vi "Access Privilege_UpdateLoginFile.vi"(8 "error in":errorcluster, 9 "Password":string, 10 "UserID":string, 11 "Cluster_In":T1) -> (0 "error out":errorcluster, 3 "Cluster_In 2":T1)   [LabVIEW 2023, in "GUI.lvlib"]
uses:
  GUI.lvlib
  Typedefs/Access Privilege_Account ManagerAppCluster.ctl
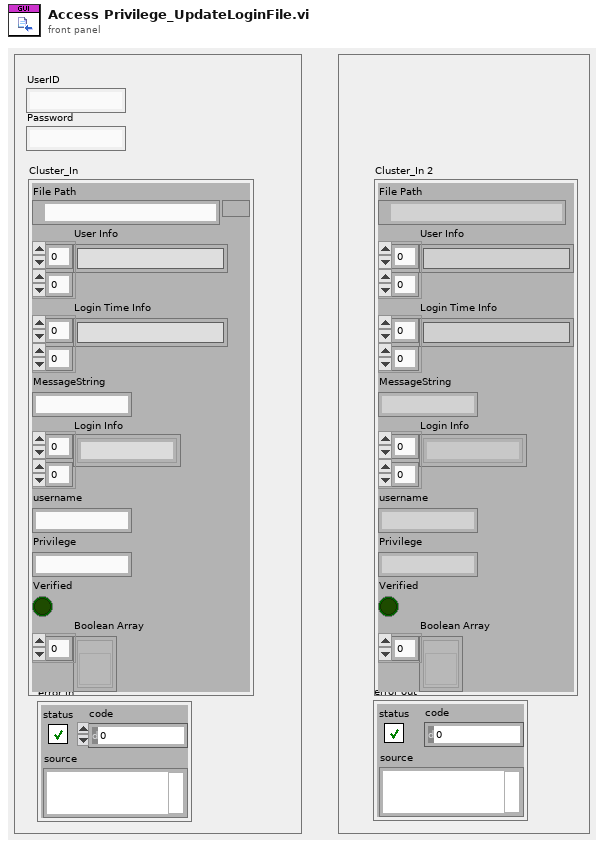
[diagram p1: front panel]
types:
  T1 = typedef "GUI.lvlib/Access Privilege_Account ManagerAppCluster.ctl" = cluster{"File Path":path, "User Info":string[][], "Login Time Info":string[][], "MessageString":string, "Login Info":string[][], "username":string, "Privilege":string, "Verified":bool, "Boolean Array":refnum<vi>[]}
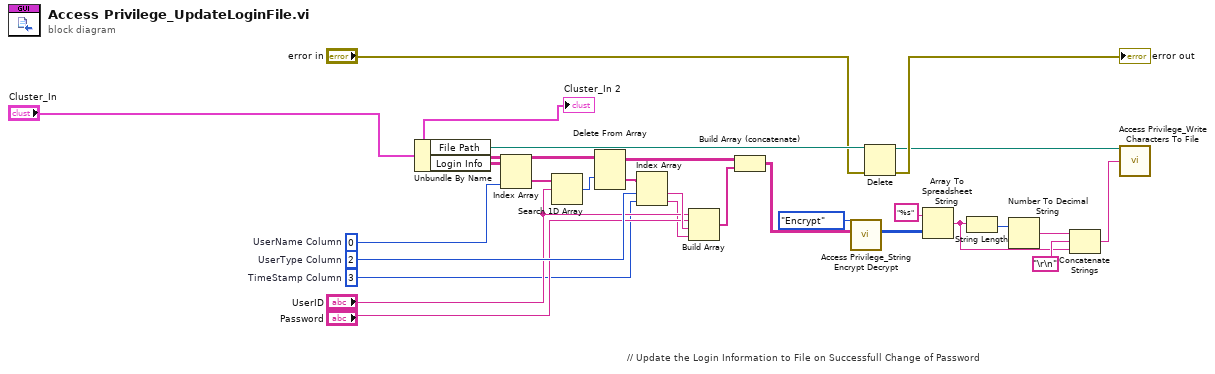
[diagram p0: block diagram]
diagram:
  w11 = 3  # TimeStamp Column
  w21 = 2  # UserType Column
  w27 = 0  # UserName Column
  # "// Update the Login Information to File on Successfull Change of Password"
  n1 = Unbundle By Name("Cluster_In") -> ("File Path"=w12:path, "Login Info"=w24:string[][])
  n2 = Index Array(array=w24, index (col)=w27) -> (element=w26:string[])  [unwired: 1 in]
  n3 = Search 1D Array(1D array=w26, element="UserID") -> (index of element=w25:i32)  [unwired: 1 out]
  n4 = Delete From Array(array=w24, index (row)=w25) -> (deleted portion=w22:string[], array with subset deleted=w23:string[][])  [unwired: 2 in]
  n5 = Index Array(array=w22, index #1=w21, index #2=w11) -> (element #1=w20:string, element #2=w10:string)
  n6 = Build Array("UserID", "Password", w20, w10) -> (w19:string[])
  n7 = Build Array (concatenate)(w23, w19) -> (w13:string[][])
  n8 = call "Access Privilege_String Encrypt Decrypt.vi"("2D String Data"=w13, "Action"=enum16{"Encrypt", "Decrypt"}."Encrypt") -> ("Encrypted Out"=w17:u8[][][])  [unwired: 8 in, 1 out]
  n9 = Delete(path (use dialog)=w12, error in="error in") -> (deleted path=w2:path, error out=→"error out":errorcluster)  [unwired: 4 out]
  n10 = Array To Spreadsheet String(array=w17, 3:"%s" ("format string")) -> (spreadsheet string=w6:string)  [unwired: 1 out]
  n11 = String Length(string=w6) -> (length=w7:i32)
  n12 = Number To Decimal String(number=w7) -> (decimal integer string=w8:string)  [unwired: 1 out]
  n13 = Concatenate Strings(w8, "\r\n", w6) -> (w5:string)
  n14 = call "Access Privilege_Write Characters To File.vi"("File path (dialog if empty)"=w2, "Character string"=w5) -> ()  [unwired: 13 in, 1 out]
  "Cluster_In 2" <- "Cluster_In"
